vi "Write Power Meter classes.vi"(10 "Power Meter classes":refnum<class "Power Meter.lvclass">[](array[class]), 11 "IMD in":refnum<class "IMD.lvclass">) -> (3 "IMD out":refnum<class "IMD.lvclass">)   [LabVIEW 2020, in "IMD.lvclass"]
uses:
  IMD.lvclass
  Instruments/Power Meter/Power Meter.lvclass
  IMD.lvclass/IMD.ctl
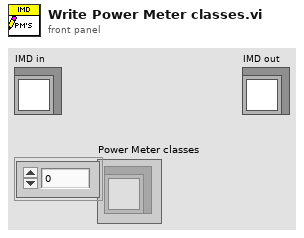
[diagram p1: front panel]
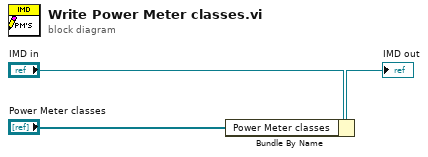
[diagram p0: block diagram]
diagram:
  n1 = Bundle By Name(cluster="IMD in", "Power Meter classes"="Power Meter classes") -> (→"IMD out":refnum<class "IMD.lvclass">)
